vi "MWT_labview_test.vi"() -> ()   [LabVIEW 2019]
uses:
  <vilib>/BLE/type_def/connection_status_bundle.ctl
  <vilib>/BLE/type_def/address_type.ctl
panel:
  in  "Connection Interval Max (95ms)":u16=95
  in  "Connection Interval Min (75ms)":u16=75
  out "Gradient graph":dbl(graph)
  out "Gradient":dbl
  out "Scanning 2":bool
  in  "Continue":bool
  in  "MAC Address":string
  in  "Address Type":T1=1 items=["Public", "Random"]
  in  "COM Bluegiga in 2":refnum<visa-resource-name>="COM13"
  out "Devices 2":string[][](array[string])
  out "BLED112 Dongle Info 2":string
  out "Rotation graph":dbl(graph)
  out "Rotation Speed":dbl
  in  "stop":bool
  out "Reading data":bool
  out "Connected":bool
  out "Device Name":string
  out "Handle table":string[][](array[string])
  out "Connection Status":T2={"MAC Address"="", "cnx handle"=0, "cnx flags"=0, "Address Type"=125, "Connection Interval (ms)"=125, "Timeout(ms)"=125, "Latency"=0, "bonding handle"=0} {"Address Type" items=["Public", "Random"]}
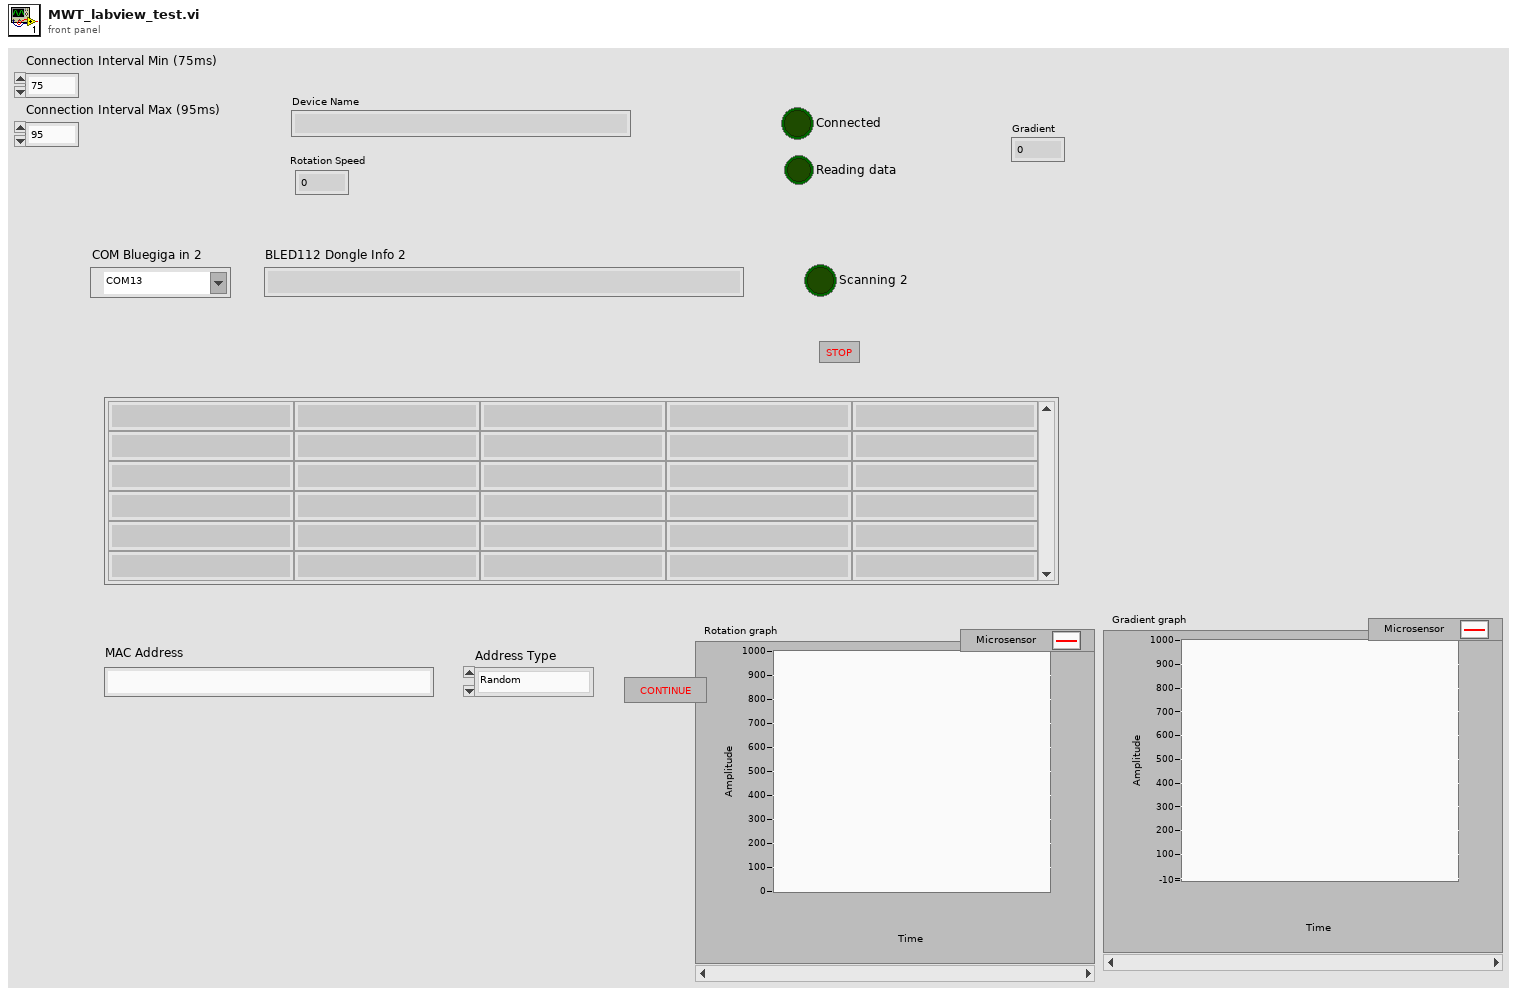
[diagram p1: front panel]
types:
  T1 = typedef "address_type.ctl" = u8
  T2 = typedef "connection_status_bundle.ctl" = cluster{"MAC Address":string, "cnx handle":u8, "cnx flags":u8, "Address Type":T1, "Connection Interval (ms)":u16, "Timeout(ms)":u16, "Latency":u16, "bonding handle":u8}
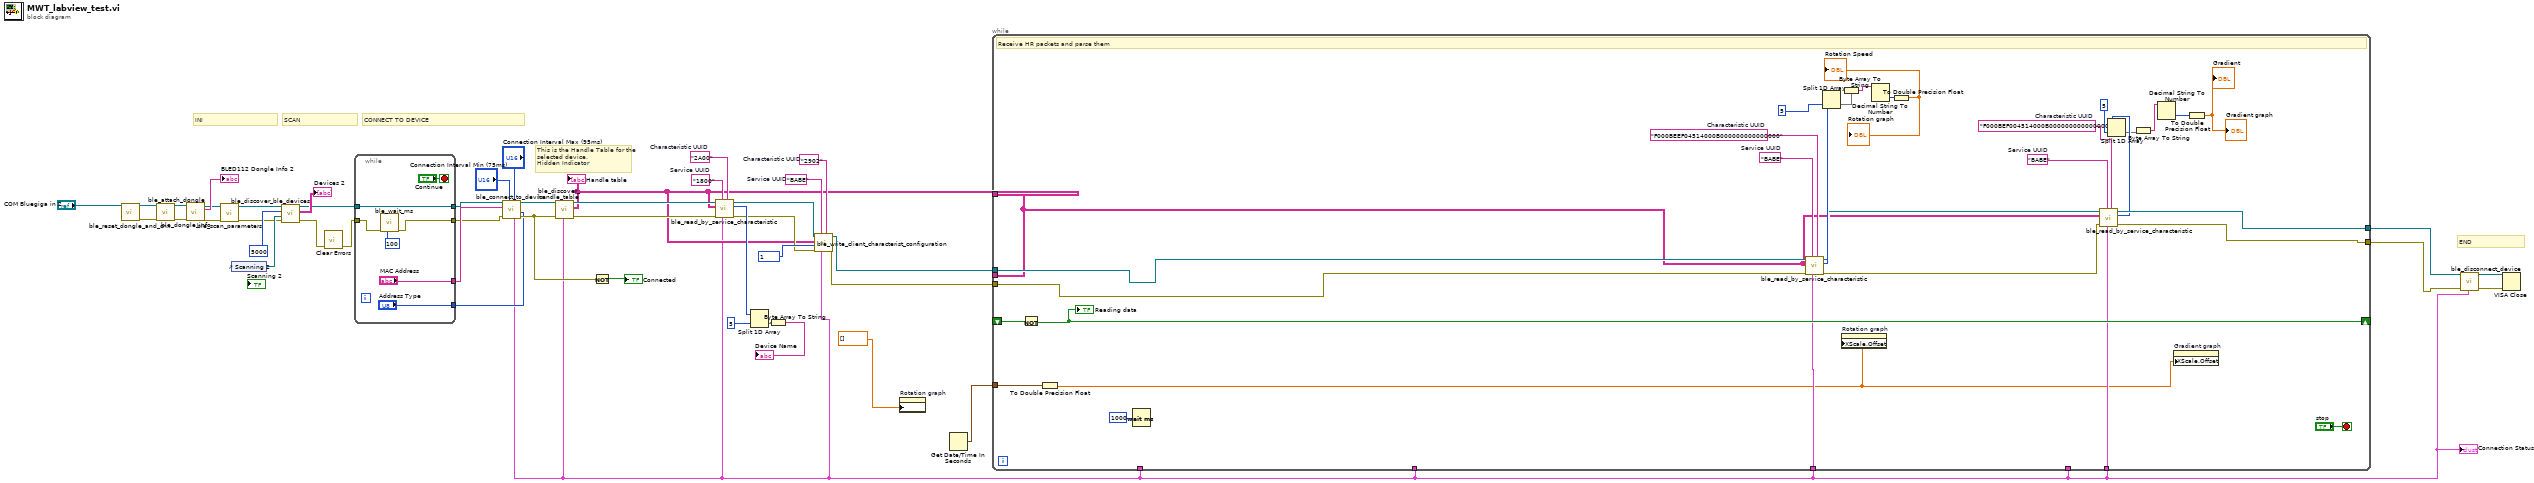
[diagram p0: block diagram]
diagram:
  w37 = "2902"  # Characteristic UUID
  w36 = "BABE"  # Service UUID
  w40 = "2A00"  # Characteristic UUID
  w41 = "1800"  # Service UUID
  # "END"
  # "This is the Handle Table for the\nselected device. \nHidden Indicator"
  # "CONNECT TO DEVICE"
  # "SCAN"
  # "INI"
  n1 = call <vilib>:"ble_reset_dongle_and_cnx.vi"("COM Bluegiga in"="COM Bluegiga in 2") -> ("error out"=w13:errorcluster, "COM Bluegiga out"=w11:refnum<visa-resource-name>)  [unwired: 9 in]
  n2 = call <vilib>:"ble_attach_dongle.vi"("error in (no error)"=w13, "COM Bluegiga in"=w11) -> ("error out"=w15:errorcluster, "COM Bluegiga out"=w14:refnum<visa-resource-name>)  [unwired: 8 in]
  n3 = call <vilib>:"ble_dongle_info.vi"("error in (no error)"=w15, "COM Bluegiga in"=w14) -> ("error out"=w18:errorcluster, "info"=→"BLED112 Dongle Info 2":string, "COM Bluegiga out"=w19:refnum<visa-resource-name>)  [unwired: 7 in]
  n4 = call <vilib>:"ble_scan_parameters.vi"("error in (no error)"=w18, "COM Bluegiga in"=w19) -> ("error out"=w16:errorcluster, "COM Bluegiga out"=w17:refnum<visa-resource-name>)  [unwired: 7 in, 1 out]
  n5 = control-ref of="Scanning 2"() -> (w20:refnum<vi>)
  n6 = call <vilib>:"ble_discover_ble_devices.vi"("error in (no error)"=w16, "LED ref"=w20, "Scan Duration (10000ms)"=u32 5000, "COM Bluegiga in"=w17) -> ("error out"=w10:errorcluster, "Devices"=→"Devices 2":string[][], "COM Bluegiga out"=w21:refnum<visa-resource-name>)  [unwired: 5 in]
  n7 = call <vilib>:"Clear Errors.vi"("error in (no error)"=w10) -> ("error out"=w9:errorcluster)  [unwired: 5 in, 1 out]
  n8 = while {
    tunnel: w9 -> [w54]
    tunnel: [w53] -> w7
    tunnel: w21 -> [w53]
    tunnel: [w52] -> w6
    tunnel: ["MAC Address"] -> w8
    tunnel: ["Address Type"] -> w5
    stop <- "Continue" stop-if-true
    n9 = call <vilib>:"ble_wait_ms.vi"("milliseconds to wait (100)"=u32 100, "error in (no error)"=w54) -> ("error out"=w52:errorcluster)  [unwired: 9 in]
  }
  n10 = call <vilib>:"ble_connect_to_device.vi"("Address Type"=w5, "Connection Interval Max (95ms)"="Connection Interval Max (95ms)", "Connection Interval Min (75ms)"="Connection Interval Min (75ms)", "error in (no error)"=w6, "MAC Address"=w8, "COM Bluegiga in"=w7) -> ("error out"=w42:errorcluster, "COM Bluegiga out"=w48:refnum<visa-resource-name>, "Connection Status"=w3:T2)  [unwired: 3 in]
  "Connection Status" <- w3
  n11 = call <vilib>:"ble_discover_handle_table.vi"("Connection Status"=w3, "error in (no error)"=w42, "COM Bluegiga in"=w48) -> ("error out"=w47:errorcluster, "Handle table"=w32:string[][], "COM Bluegiga out"=w46:refnum<visa-resource-name>)  [unwired: 6 in]
  "Handle table" <- w32
  n12 = Not(x=w42) -> (.not. x?=→"Connected":bool)
  n13 = call <vilib>:"ble_read_by_service_characteristic.vi"("Characteristic UUID"=w40, "Connection Status"=w3, "Service UUID"=w41, "error in (no error)"=w47, "Handle table"=w32, "COM Bluegiga in"=w46) -> ("error out"=w33:errorcluster, "characteristic value"=w39:u8[], "COM Bluegiga out"=w34:refnum<visa-resource-name>)  [unwired: 3 in]
  n14 = Split 1D Array(array=w39, index=5) -> (second subarray=w38:u8[])  [unwired: 1 out]
  n15 = Byte Array To String(unsigned byte array=w38) -> (string=→"Device Name":string)
  n16 = call <vilib>:"ble_write_client_characterist_configuration.vi"("Characteristic UUID"=w37, "Connection Status"=w3, "Service UUID"=w36, "error in (no error)"=w33, "Value(16bit)"=u16 1, "Handle table"=w32, "COM Bluegiga in"=w34) -> ("error out"=w30:errorcluster, "COM Bluegiga out"=w31:refnum<visa-resource-name>)  [unwired: 3 in]
  n17 = property on="Rotation graph" class="WFChart (strict)"("History Data"=dbl[] []) -> ()  [unwired: 2 in, 2 out]
  n18 = Get Date/Time In Seconds() -> (seconds since 1Jan1904=w4:timestamp)
  n19 = while {
    shift-right: [w78] -> _
    shift-left: _ -> [w85]
    tunnel: [w58] -> _
    tunnel: w32 -> [w58]
    tunnel: w3 -> [w77]
    tunnel: w31 -> [w74]
    tunnel: w30 -> [w73]
    tunnel: [w64] -> w27
    tunnel: [w63] -> w28
    tunnel: w3 -> [_]
    tunnel: w3 -> [_]
    tunnel: w3 -> [_]
    tunnel: w4 -> [w72]
    tunnel: w3 -> [w57]
    stop <- "stop" stop-if-true
    w62 = "F000BEF004514000B000000000000000"  # Characteristic UUID
    w61 = "BABE"  # Service UUID
    w83 = "F000BEEF04514000B000000000000000"  # Characteristic UUID
    w84 = "BABE"  # Service UUID
    # "Receive HR packets and parse them"
    n20 = Not(x=w85) -> (.not. x?=w78:bool)
    "Reading data" <- w78
    n21 = To Double Precision Float(number=w72) -> (double precision float=w56:dbl)
    n22 = Wait (ms)(milliseconds to wait=u32 1000) -> ()  [unwired: 1 out]
    n23 = call <vilib>:"ble_read_by_service_characteristic.vi"("Characteristic UUID"=w83, "Connection Status"=w77, "Service UUID"=w84, "error in (no error)"=w73, "Handle table"=w58, "COM Bluegiga in"=w74) -> ("error out"=w65:errorcluster, "characteristic value"=w75:u8[], "COM Bluegiga out"=w66:refnum<visa-resource-name>)  [unwired: 3 in]
    n24 = Split 1D Array(array=w75, index=5) -> (second subarray=w81:u8[])  [unwired: 1 out]
    n25 = property on="Rotation graph" class="WFChart (strict)"("XScale.Offset"=w56) -> ()  [unwired: 2 in, 2 out]
    n26 = Byte Array To String(unsigned byte array=w81) -> (string=w80:string)
    n27 = Decimal String To Number(string=w80) -> (number=w79:i32)  [unwired: 2 in, 1 out]
    n28 = To Double Precision Float(number=w79) -> (double precision float=→"Rotation Speed" →"Rotation graph":dbl)
    n29 = call <vilib>:"ble_read_by_service_characteristic.vi"("Characteristic UUID"=w62, "Connection Status"=w57, "Service UUID"=w61, "error in (no error)"=w65, "Handle table"=w58, "COM Bluegiga in"=w66) -> ("error out"=w64:errorcluster, "characteristic value"=w60:u8[], "COM Bluegiga out"=w63:refnum<visa-resource-name>)  [unwired: 3 in]
    n30 = Split 1D Array(array=w60, index=5) -> (second subarray=w59:u8[])  [unwired: 1 out]
    n31 = Byte Array To String(unsigned byte array=w59) -> (string=w68:string)
    n32 = Decimal String To Number(string=w68) -> (number=w69:i32)  [unwired: 2 in, 1 out]
    n33 = property on="Gradient graph" class="WFChart (strict)"("XScale.Offset"=w56) -> ()  [unwired: 2 in, 2 out]
    n34 = To Double Precision Float(number=w69) -> (double precision float=→"Gradient" →"Gradient graph":dbl)
  }
  n35 = call <vilib>:"ble_disconnect_device.vi"("Connection Status"=w3, "error in (no error)"=w27, "COM Bluegiga in"=w28) -> ("error out"=w25:errorcluster, "COM Bluegiga out"=w26:refnum<visa-resource-name>)  [unwired: 7 in]
  n36 = VISA Close(VISA resource name=w26, error in (no error)=w25) -> ()  [unwired: 1 out]
